vi "Math_Reciprocal.vi"(1 "x":fxp<+/-,32,16> format="%#_32g") -> (0 "1/x":fxp<+/-,32,16>)   [LabVIEW 2020]
uses:
  <vilib>/rvi/FXPMathLib/FxpReciprocal/XNode/nifxpmath_Reciprocal.xnode
  <vilib>/rvi/FXPMathLib/FxpDiv/XNode/nifxpmath_Div.xnode
  <vilib>/rvi/FXPMathLib/FxpDiv/simVIs/DllFxpDivTemp_sub.vi
  <vilib>/rvi/FXPMathLib/FxpDiv/subVIs/nifxpmath_Div_SimConfig.ctl
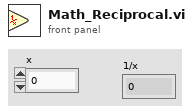
[diagram p1: front panel]
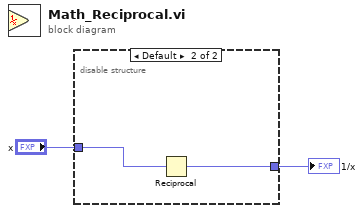
[diagram p0: block diagram]
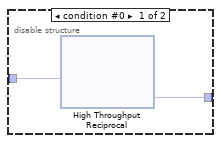
[diagram p2: hidden frame]
diagram:
  n1 = disable-structure shown="Default" {
    disable-tunnel: "x" -> [w4 w36]
    disable-tunnel: [w3 w35] -> w1
    frame condition #0 {
      n2 = xnode "High Throughput Reciprocal"("x"=w4) -> ("1/x"=w3:fxp<+/-,32,16>)
    }
    frame condition #1 (active) {
      n3 = Reciprocal(x=w36) -> (1/x=w35:fxp<+/-,32,16>)
    }
  }
  "1/x" <- w1
